vi "Z900_navX_SERIAL_DecodePacket.vi"(8 "error in (no error)":errorcluster, 10 "Data":u8[](array[numeric]), 11 "Packet":string) -> (0 "error out":errorcluster, 2 "Data":u8[](array[numeric]), 3 "Packet":string)   [LabVIEW 2014, in "navX Library v2.lvlib"]
uses:
  navX Library v2.lvlib
  TypeDefs/Z900_navX_DeviceRegisters.ctl
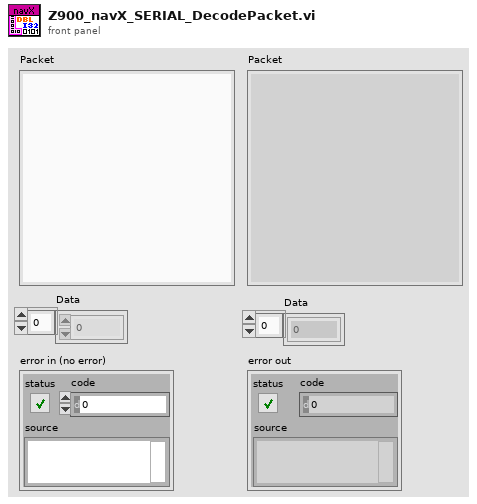
[diagram p1: front panel]
types:
  T1 = typedef "navX Library v2.lvlib/Z900_navX_DeviceRegisters.ctl" = u8
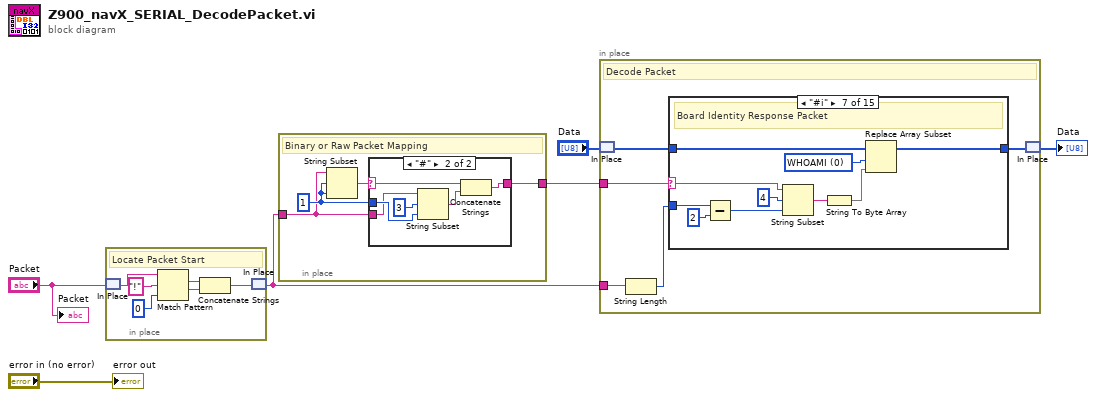
[diagram p0: block diagram]
diagram:
  n1 = in-place {
    # "Locate Packet Start"
    n2 = in-place-match #1("Packet") -> (w8:string)
    n3 = Match Pattern(string=w8, regular expression="!" ("Packet Start Char"), offset (0)=0 ("offset past match")) -> (match substring=w11:string, after substring=w10:string)  [unwired: 2 out]
    n4 = Concatenate Strings(w11, w10) -> (w7:string)
    n5 = in-place-match #1(w7) -> (w2:string)
  }
  n6 = in-place {
    in-place-border: w2 -> [w14]
    in-place-border: [w16] -> w3
    w15 = 1 ("length (rest)")
    # "Binary or Raw Packet Mapping"
    n7 = String Subset(string=w14, offset (0)=w15, length (rest)=w15) -> (substring=w13:string)
    n8 = case shown="\"#\"" w13 {
      selector: w13 -> [w17 w18]
      tunnel: [w17 w19] -> w16
      tunnel: w15 -> [_ w22]
      tunnel: w14 -> [_ w21]
      frame Default {
      }
      frame "#" {
        n9 = String Subset(string=w21, offset (0)=3, length (rest)=w22) -> (substring=w20:string)
        n10 = Concatenate Strings(w18, w20) -> (w19:string)
      }
    }
  }
  n11 = in-place {
    in-place-border: w3 -> [w27]
    in-place-border: w2 -> [w28]
    # "Decode Packet"
    n12 = in-place-match #2("Data") -> (w25:u8[])
    n13 = String Length(string=w28) -> (length=w26:i32)
    n14 = case shown="\"#i\"" w27 {
      selector: w27 -> [_ _ _ _ _ _ w44 _ _ _ _ _ _ _ _]
      tunnel: w26 -> [_ _ _ _ _ _ w42 _ _ _ _ _ _ _ _]
      tunnel: w25 -> [w29 w30 w31 w32 w33 w34 w38 w45 w46 w47 w48 w49 w50 w51 w52]
      tunnel: [w29 w30 w31 w32 w33 w34 w35 w45 w46 w47 w48 w49 w50 w51 w52] -> w24
      frame Default {
        # "We should not care about decoding this packet type."
        # "Unknown Packet"
      }
      frame "y" {
        # "Yaw/Pitch/Roll (YPR) Update Packet"
      }
      frame "q" {
        # "Quaternion Update Packet"
      }
      frame "g" {
        # "Gyro/Raw Data Update Packet"
      }
      frame "s" {
        # "EnableStream Response Packet"
      }
      frame "#a" {
        # "AHRS Update Packet"
      }
      frame "#i" {
        w37 = T1 0 items=["WHOAMI"=0, "HW_REV"=1, "FW_VER_MAJOR"=2, "FW_VER_MINOR"=3, "UPDATE_RATE_HZ"=4, "ACCEL_FSR_G"=5, "GYRO_FSR_DPS"=6, "OP_STATUS"=8, "CAL_STATUS"=9, "SELFTEST_STATUS"=10, "CAPABILITY_FLAGS_L"=11, "CAPABILITY_FLAGS_H"=12, "SENSOR_STATUS"=16, "TIMESTAMP"=18, "YAW"=22, "ROLL"=24, "PITCH"=26, "HEADING"=28, "FUSED_HEADING"=30, "ALTITUDE_I"=32, "ALTITUDE_D"=34, "LINERA_ACC_X"=36, "LINERA_ACC_Y"=38, "LINERA_ACC_Z"=40, "QUAT_W"=42, "QUAT_X"=44, "QUAT_Y"=46, "QUAT_Z"=48, "MPU_TEMP_C"=50, "GYRO_X"=52, "GYRO_Y"=54, "GYRO_Z"=56, "ACC_X"=58, "ACC_Y"=60, "ACC_Z"=62, "MAG_X"=64, "MAG_Y"=66, "MAG_Z"=68, "PRESSURE_I"=70, "PRESSURE_D"=72, "PRESSURE_TEMP"=74, "YAW_OFFSET"=76, "QUAT_OFFSET_W"=78, "QUAT_OFFSET_X"=80, "QUAT_OFFSET_Y"=82, "QUAT_OFFSET_Z"=84, "INTEGRATION_CONTROL"=86, "VELOCITY_X"=88, "VELOCITY_Y"=92, "VELOCITY_Z"=96, "DISPLACMENT_X"=100, "DISPLACMENT_Y"=104, "DISPLACEMENT_Z"=108] ("Device Register")
        # "Board Identity Response Packet"
        n15 = Subtract(x=w42, y=2) -> (x-y=w40:i32)
        n16 = String Subset(string=w44, offset (0)=4, length (rest)=w40) -> (substring=w39:string)
        n17 = String To Byte Array(string=w39) -> (unsigned byte array=w36:u8[])
        n18 = Replace Array Subset(array=w38, new element=w36, index=w37) -> (w35:u8[])
      }
      frame "#j" {
        # "Integration Control Response Packet"
      }
      frame "#p" {
        # "AHRSAndPositioning Update Packet"
      }
      frame "#v" {
        # "Data Set Response Packet"
      }
      frame "S" {
        # "We should not care about decoding this packet type."
        # "EnableStream Command Packet"
      }
      frame "#D" {
        # "We should not care about decoding this packet type."
        # "Data Get Request"
      }
      frame "#I" {
        # "We should not care about decoding this packet type."
        # "Integration Control Command Packet"
      }
      frame "#M" {
        # "We should not care about decoding this packet type."
        # "Magnetometer Calibration Packet"
      }
      frame "#T" {
        # "We should not care about decoding this packet type."
        # "Tuning Variable Packet"
      }
    }
    n19 = in-place-match #2(w24) -> (→"Data":u8[])
  }
  "Packet" <- "Packet"
  "error out" <- "error in (no error)"
